vi "Handle Error.vi"(8 "error in (no error)":errorcluster, 11 "Command Processor Actor in":refnum<class "Command Processor Actor.lvclass">) -> (0 "error out":errorcluster, 2 "stop actor?":bool=TRUE, 3 "Command Processor Actor out":refnum<class "Command Processor Actor.lvclass">)   [LabVIEW 2014, in "Robot Actor Framework.lvlib" / "Command Processor Actor.lvlib" / "Command Processor Actor.lvclass"]
doc: "(<B>Filename</B>: Actor Framework.lvlib:Actor.lvclass:Handle Error.vi)\n\nDefines how the actor handles an error that occurred while processing a message. By default, this method does nothing except stop the actor."
uses:
  Command Processor Actor.lvclass
  <vilib>/ni/Actors/State Actor/State Actor/State Actor.lvclass
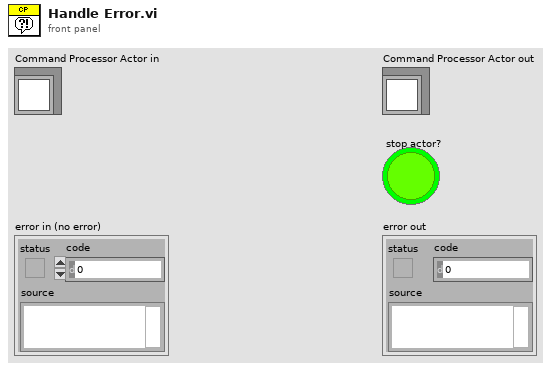
[diagram p1: front panel]
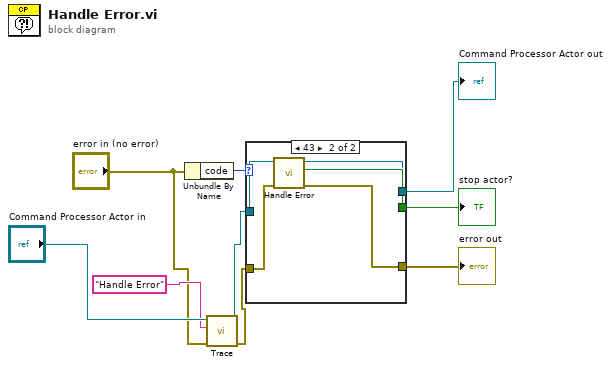
[diagram p0: block diagram]
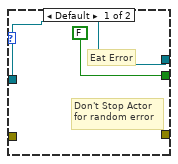
[diagram p2: hidden frame]
diagram:
  n1 = Unbundle By Name("error in (no error)") -> ("code"=w6:i32)
  n2 = call-dynamic "Trace.vi"("error in (no error)"="error in (no error)", "Command Processor Action"="Handle Error" ("Command Processor Message"), "Command Processor Actor in"="Command Processor Actor in") -> ("error out"=w1:errorcluster, "Command Processor Actor out"=w2:refnum<class "Command Processor Actor.lvclass">)  [unwired: 7 in]
  n3 = case shown="43" w6 {
    tunnel: [_ w16] -> w9
    tunnel: [FALSE ("stop actor?") w15] -> w8
    tunnel: [w10 w14] -> w7
    tunnel: w2 -> [w10 w13]
    tunnel: w1 -> [_ w12]
    frame Default {
      # "Don't Stop Actor\nfor random error"
      # "Eat Error"
    }
    frame 43 {
      n4 = call-parent "Handle Error.vi"("error in (no error)"=w12, "Actor in"=w13) -> ("error out"=w16:errorcluster, "stop actor?"=w15:bool, "Actor out"=w14:refnum<class "Command Processor Actor.lvclass">)  [unwired: 7 in]
    }
  }
  "Command Processor Actor out" <- w7
  "error out" <- w9
  "stop actor?" <- w8
